vi "Ultimus.vi"   [LabVIEW 2016]
uses:
  Classes/Controllers/Dispenser/Copy of Ultimus V2 Folder/Ultimus V2.lvclass
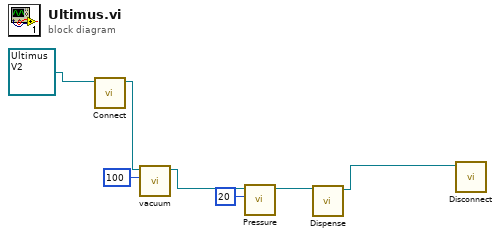
[diagram p0: block diagram]
diagram:
  n1 = call-dynamic "Connect.vi"("Ultimus V in"=refnum<class "Ultimus V2.lvclass"> refnum ("Ultimus V2.lvclass")) -> ("Ultimus V out"=w6:refnum<class "Ultimus V2.lvclass">)  [unwired: 9 in, 1 out]
  n2 = call "vacuum.vi"("Vacuum Setting (0000)"=i64 100, "Ultimus V in"=w6) -> ("Ultimus V out"=w5:refnum<class "Ultimus V2.lvclass">)  [unwired: 8 in, 1 out]
  n3 = call-dynamic "Pressure.vi"("Pressure"=i16 20, "Ultimus V in"=w5) -> ("Ultimus V out"=w4:refnum<class "Ultimus V2.lvclass">)  [unwired: 8 in, 1 out]
  n4 = call-dynamic "Dispense.vi"("Ultimus V in"=w4) -> ("Ultimus V out"=w3:refnum<class "Ultimus V2.lvclass">)  [unwired: 9 in, 1 out]
  n5 = call-dynamic "Disconnect.vi"("Ultimus V in"=w3) -> ()  [unwired: 9 in, 1 out]
